vi "打开Excel.vi"(8 "错误输入（无错误）":errorcluster, 10 "文件路径":path, 11 "Excel._Application":refnum<k7>) -> (0 "错误输出":errorcluster, 3 "引用簇":T1)   [LabVIEW 2021, in "OperateExcel.lvlib"]
uses:
  OperateExcel.lvlib
  <vilib>/Utility/error.llb/Error Cluster From Error Code.vi
  <vilib>/ErrorRing/Error Ring.xnode
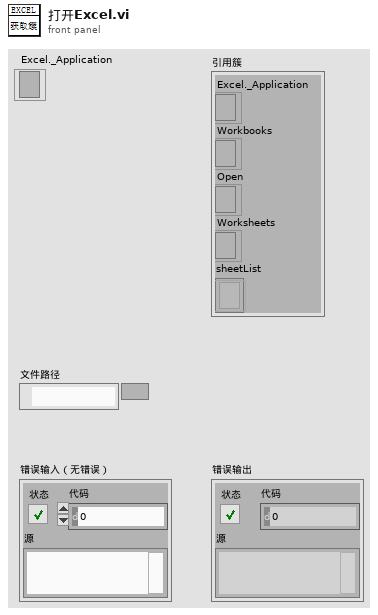
[diagram p1: front panel]
types:
  T1 = typedef "OperateExcel.lvlib/引用簇.ctl" = cluster{"Excel._Application":refnum<k7>, "Workbooks":refnum<k7>, "Open":refnum<k7>, "Worksheets":refnum<k7>, "sheetList":refnum<k7>[]}
  T2 = enum32{"invalid app kind", "Development System", "Run Time System", "Student Edition", "Embedded LabVIEW", "Evaluation", "Custom"}
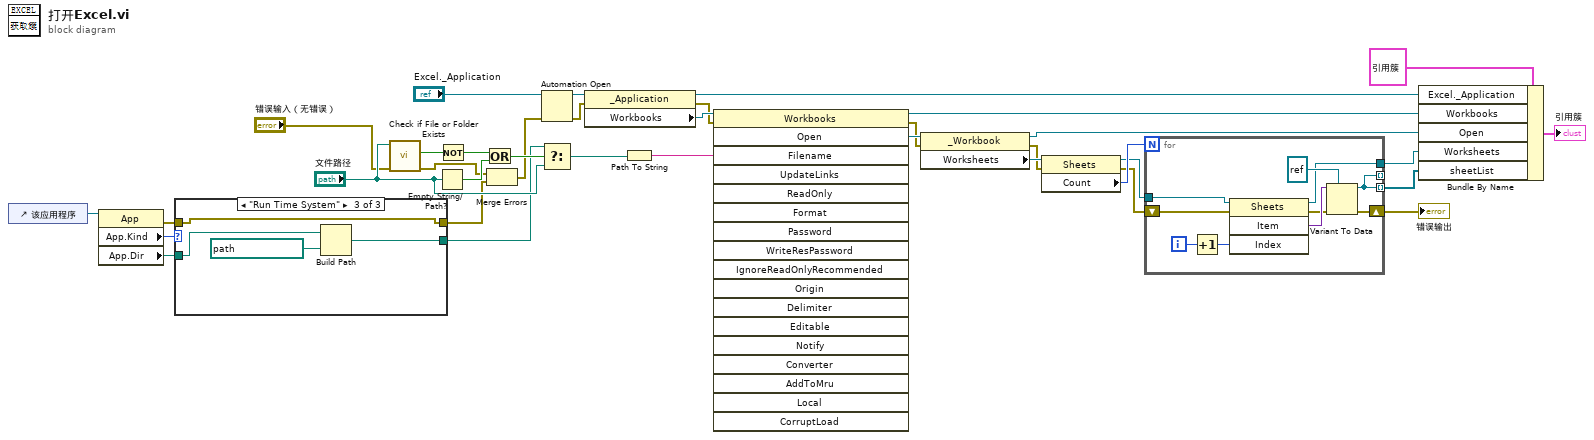
[diagram p0: block diagram]
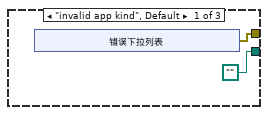
[diagram p2: hidden frame]
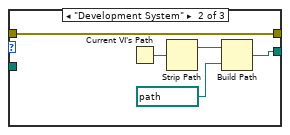
[diagram p3: hidden frame]
diagram:
  n1 = control-ref of="该应用程序"() -> (w9:refnum<vi>)
  n2 = property class="App"(reference=w9) -> (error out=w5:errorcluster, "App.Kind"=w8:T2, "App.Dir"=w7:path)  [unwired: 1 in, 1 out]
  n3 = case shown="\"Run Time System\"" w8 {
    tunnel: w7 -> [_ _ w50]
    tunnel: [path "" w44 w49] -> w6
    tunnel: w5 -> [_ w43 w48]
    tunnel: [w38 w43 w48] -> w3
    frame "invalid app kind", Default {
      n4 = xnode "错误下拉列表"() -> ("错误输出"=w38:errorcluster)
    }
    frame "Development System" {
      n5 = Current VI's Path() -> (path=w46:path)
      n6 = Strip Path(path=w46) -> (stripped path=w47:path)  [unwired: 1 out]
      n7 = Build Path(base path=w47, name or relative path=path "模板.xlsx" ("文件路径")) -> (appended path=w44:path)
    }
    frame "Run Time System" {
      n8 = Build Path(base path=w50, name or relative path=path "data/模板.xlsx" ("文件路径")) -> (appended path=w49:path)
    }
  }
  n9 = call <vilib>:"Check if File or Folder Exists.vi"("error in (no error)"="错误输入（无错误）", "path"="文件路径") -> ("error out"=w2:errorcluster, "file or folder exists?"=w11:bool)  [unwired: 7 in, 1 out]
  n10 = Empty String/Path?(string/path="文件路径") -> (empty?=w13:bool)
  n11 = Not(x=w11) -> (.not. x?=w10:bool)
  n12 = Or(x=w10, y=w13) -> (x .or. y?=w12:bool)
  n13 = Merge Errors(w2, w3) -> (w1:errorcluster)
  n14 = Automation Open(error in (no error)=w1, Automation Refnum="Excel._Application") -> (Automation Refnum=w18:refnum<k7>, error out=w17:errorcluster)  [unwired: 2 in]
  n15 = Select(t=w6, s=w12, f="文件路径") -> (s? t:f=w15:path)
  n16 = property class="_Application"(reference=w18, error in=w17) -> (reference out=w25:refnum<k7>, error out=w33:errorcluster, "Workbooks"=w36:refnum<k7>)
  n17 = Path To String(path=w15) -> (string=w35:string)
  n18 = invoke class="Workbooks" method="Open"(reference=w36, error in=w33, "Filename"=w35) -> (reference out=w24:refnum<k7>, error out=w32:errorcluster, "Open"=w34:refnum<k7>)  [unwired: 15 in, 15 out]
  n19 = property class="_Workbook"(reference=w34, error in=w32) -> (reference out=w23:refnum<k7>, error out=w30:errorcluster, "Worksheets"=w31:refnum<k7>)
  n20 = property class="Sheets"(reference=w31, error in=w30) -> (reference out=w28:refnum<k7>, error out=w27:errorcluster, "Count"=w29:i32)
  n21 = for {
    N: w29 -> [_]
    tunnel: w28 -> [w61]
    tunnel: [w52] -> _ mode=indexing
    shift-right: [w54] -> w26
    shift-left: w27 -> [w60]
    tunnel: [w53] -> w22
    tunnel: [w52] -> w21 mode=indexing
    i -> [w59]
    n22 = Increment(x=w59) -> (x+1=w58:i32)
    n23 = invoke class="Sheets" method="Item"(reference=w61, error in=w60, "Index"=w58) -> (reference out=w53:refnum<k7>, error out=w55:errorcluster, "Item"=w57:variant)  [unwired: 1 in, 1 out]
    n24 = Variant To Data(error in=w55, type=refnum<k7> refnum ("引用输出"), Variant=w57) -> (data=w52:refnum<k7>, error out=w54:errorcluster)
  }
  "错误输出" <- w26
  n25 = Bundle By Name(cluster=T1 {"Excel._Application"=refnum, "Workbooks"=refnum, "Open"=refnum, "Worksheets"=refnum, "sheetList"=[refnum]} ("引用簇"), "Excel._Application"=w25, "Workbooks"=w24, "Open"=w23, "Worksheets"=w22, "sheetList"=w21) -> (→"引用簇":T1)
